vi "AudioTest.Get UUT Result Info.vi"(11 "Folder":path) -> (1 "Misc Data":string[][](array[string]), 3 "Result":string[](array[string]))   [LabVIEW 2018]
uses:
  <vilib>/KATE/Files/File Utils.lvlib
panel:
  # "State\nCode\nDesc\nLocation"
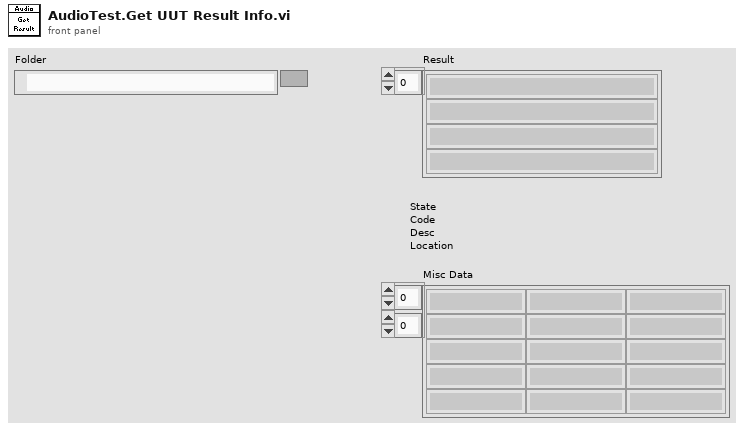
[diagram p1: front panel]
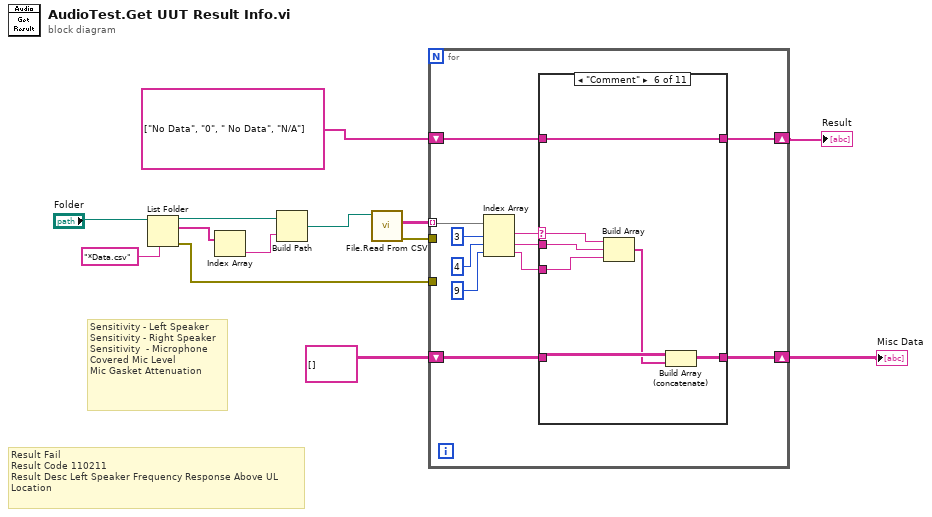
[diagram p0: block diagram]
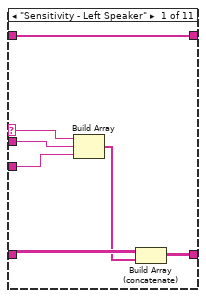
[diagram p2: hidden frame]
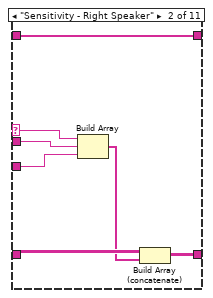
[diagram p3: hidden frame]
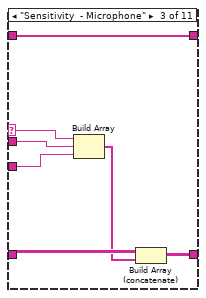
[diagram p4: hidden frame]
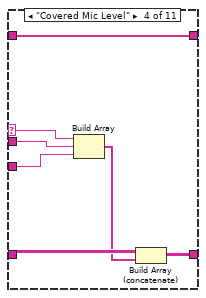
[diagram p5: hidden frame]
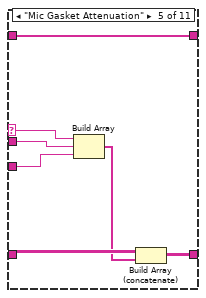
[diagram p6: hidden frame]
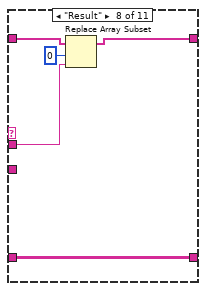
[diagram p8: hidden frame]
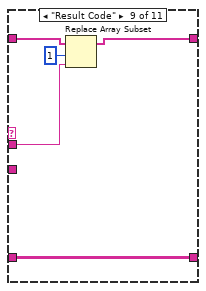
[diagram p9: hidden frame]
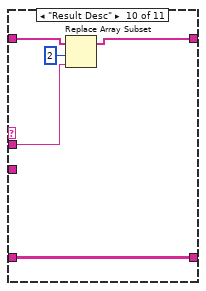
[diagram p10: hidden frame]
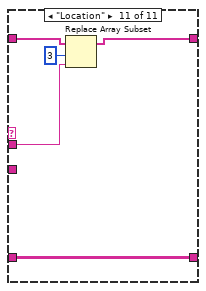
[diagram p11: hidden frame]
diagram:
  # "Sensitivity - Left Speaker\nSensitivity - Right Speaker\nSensitivity  - Microphone\nCovered Mic Level\nMic Gasket Attenuation"
  # "Result\tFail\nResult Code\t110211\nResult Desc\tLeft Speaker Frequency Response Above UL\nLocation"
  n1 = List Folder(path="Folder", pattern="*Data.csv") -> (path out=w10:path, filenames=w11:string[], error out=w3:errorcluster)  [unwired: 2 in, 1 out]
  n2 = Index Array(array=w11) -> (element=w9:string)  [unwired: 1 in]
  n3 = Build Path(base path=w10, name or relative path=w9) -> (appended path=w8:path)
  n4 = call <vilib>:"File.Read From CSV.vi"("File"=w8) -> ("error out"=w4:errorcluster, "Data"=w7:string[][])  [unwired: 8 in, 1 out]
  n5 = for {
    tunnel: w7 -> [w24] mode=indexing
    shift-right: [w19] -> w5
    shift-left: string[] ["No Data", "0", " No Data", "N/A"] -> [w20]
    tunnel: w4 -> [_]
    tunnel: w3 -> [_]
    shift-right: [w14] -> w1
    shift-left: string[][] [] -> [w17]
    n6 = Index Array(array=w24, index #1=3 ("index"), index #2=4 ("index"), index #3=9 ("index")) -> (element #1=w22:string, element #2=w21:string, element #3=w15:string)
    n7 = case shown="\"Comment\"" w22 {
      selector: w22 -> [w30 w37 w44 w51 w58 w65 _ _ _ _ _]
      tunnel: w21 -> [w29 w36 w43 w50 w57 w64 _ w72 w77 w82 w87]
      tunnel: w20 -> [w31 w38 w45 w52 w59 w66 w68 w73 w78 w83 w88]
      tunnel: [w31 w38 w45 w52 w59 w66 w68 w71 w76 w81 w86] -> w19
      tunnel: w17 -> [w26 w33 w40 w47 w54 w61 w67 w69 w74 w79 w84]
      tunnel: w15 -> [w28 w35 w42 w49 w56 w63 _ _ _ _ _]
      tunnel: [w27 w34 w41 w48 w55 w62 w67 w69 w74 w79 w84] -> w14
      frame "Sensitivity - Left Speaker" {
        n8 = Build Array(w30, w29, w28) -> (w25:string[])
        n9 = Build Array (concatenate)(w26, w25) -> (w27:string[][])
      }
      frame "Sensitivity - Right Speaker" {
        n10 = Build Array(w37, w36, w35) -> (w32:string[])
        n11 = Build Array (concatenate)(w33, w32) -> (w34:string[][])
      }
      frame "Sensitivity  - Microphone" {
        n12 = Build Array(w44, w43, w42) -> (w39:string[])
        n13 = Build Array (concatenate)(w40, w39) -> (w41:string[][])
      }
      frame "Covered Mic Level" {
        n14 = Build Array(w51, w50, w49) -> (w46:string[])
        n15 = Build Array (concatenate)(w47, w46) -> (w48:string[][])
      }
      frame "Mic Gasket Attenuation" {
        n16 = Build Array(w58, w57, w56) -> (w53:string[])
        n17 = Build Array (concatenate)(w54, w53) -> (w55:string[][])
      }
      frame "Comment" {
        n18 = Build Array(w65, w64, w63) -> (w60:string[])
        n19 = Build Array (concatenate)(w61, w60) -> (w62:string[][])
      }
      frame Default {
      }
      frame "Result" {
        n20 = Replace Array Subset(array=w73, new element=w72, index=0) -> (w71:string[])
      }
      frame "Result Code" {
        n21 = Replace Array Subset(array=w78, new element=w77, index=1) -> (w76:string[])
      }
      frame "Result Desc" {
        n22 = Replace Array Subset(array=w83, new element=w82, index=2) -> (w81:string[])
      }
      frame "Location" {
        n23 = Replace Array Subset(array=w88, new element=w87, index=3) -> (w86:string[])
      }
    }
  }
  "Result" <- w5
  "Misc Data" <- w1
